vi "GetYawPitchRollCompass.vi"(0 "Nav6DevRef":T1, 5 "error in (no error)":errorcluster) -> (12 "Yaw (Raw)":dbl, 14 "Nav6DevRef Out":T1, 15 "Yaw":dbl, 16 "Pitch":dbl, 17 "Roll":dbl, 18 "Compass Heading":dbl, 19 "error out":errorcluster)   [LabVIEW 2013, in "Nav6.lvlib"]
uses:
  Nav6.lvlib
  Nav6DevRef.ctl
  <vilib>/Rock Robotics/WPI/SerialPort/WPI_SerialPortRef.ctl
  Nav6Mode.ctl
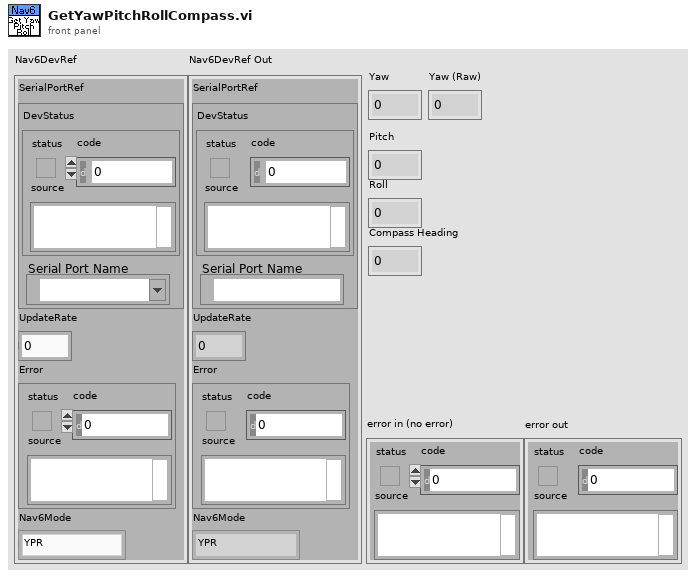
[diagram p1: front panel]
types:
  T1 = typedef "Nav6.lvlib/Nav6DevRef.ctl" = cluster{"SerialPortRef":T2, "UpdateRate":u8, "Error":errorcluster, "Nav6Mode":T3}
  T2 = typedef "WPI_SerialPortRef.ctl" = cluster{"DevStatus":errorcluster, "Serial Port Name":refnum<visa-resource-name>}
  T3 = typedef "Nav6.lvlib/Nav6Mode.ctl" = enum16{"YPR", "Gyro", "Quaternion"}
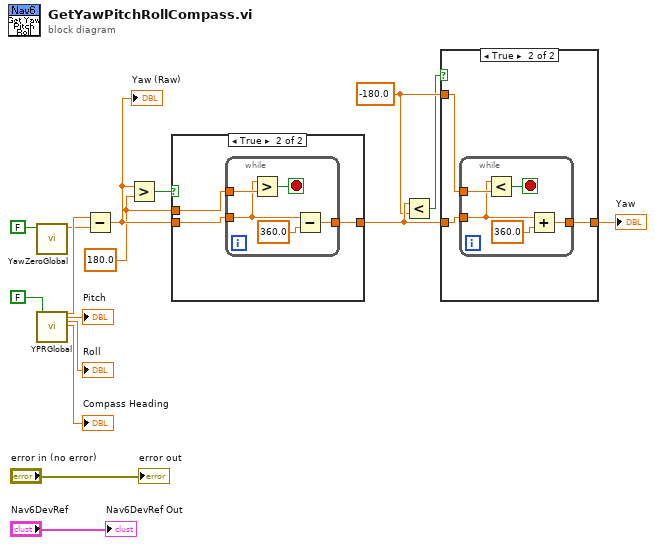
[diagram p0: block diagram]
diagram:
  w7 = -180.0 ("y")
  w12 = 180.0 ("y")
  n1 = call "YawZeroGlobal.vi"("Update"=FALSE) -> ("YawZero"=w14:dbl)  [unwired: 10 in]
  n2 = call "YPRGlobal.vi"("Update"=FALSE) -> ("Yaw Out"=w15:dbl, "Pitch Out"=→"Pitch":dbl, "Roll Out"=→"Roll":dbl, "Compass Heading Out"=→"Compass Heading":dbl)  [unwired: 20 in, 3 out]
  n3 = Subtract(x=w15, y=w14) -> (x-y=w13:dbl)
  "Yaw (Raw)" <- w13
  n4 = Greater?(x=w13, y=w12) -> (0:w9:bool)
  n5 = case shown="True" w9 {
    tunnel: w13 -> [w17 w20]
    tunnel: [w17 w18] -> w8
    tunnel: w12 -> [_ w19]
    frame False {
    }
    frame True {
      n6 = while {
        tunnel: w20 -> [w22]
        tunnel: w19 -> [w24]
        tunnel: [w23] -> w18
        stop <- w25 stop-if-true
        n7 = Greater?(x=w22, y=w24) -> (0:w25:bool)
        n8 = Subtract(x=w22, y=360.0) -> (x-y=w23:dbl)
      }
    }
  }
  n9 = Less?(x=w8, y=w7) -> (x < y?=w6:bool)
  n10 = case shown="True" w6 {
    tunnel: w8 -> [w26 w29]
    tunnel: [w26 w27] -> w11
    tunnel: w7 -> [_ w28]
    frame False {
    }
    frame True {
      n11 = while {
        tunnel: w29 -> [w31]
        tunnel: w28 -> [w33]
        tunnel: [w32] -> w27
        stop <- w34 stop-if-true
        n12 = Less?(x=w31, y=w33) -> (x < y?=w34:bool)
        n13 = Add(x=w31, y=360.0) -> (x+y=w32:dbl)
      }
    }
  }
  "Yaw" <- w11
  "Nav6DevRef Out" <- "Nav6DevRef"
  "error out" <- "error in (no error)"
